vi "FT10_Wait Minimum Milliseconds.vi"(7 "Minimum ms wait":u32, 8 "error in (no error)":errorcluster, 11 "previous millisecond timer value in":u32) -> (0 "error out":errorcluster, 3 "millisecond timer value out":u32)   [LabVIEW 2015]
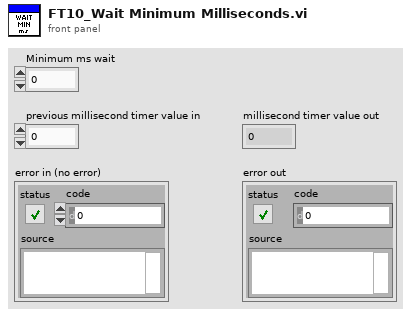
[diagram p1: front panel]
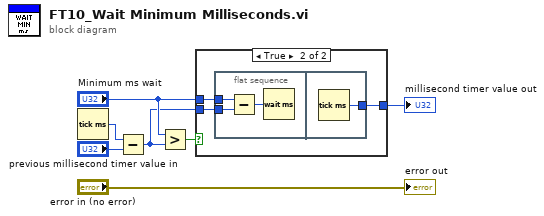
[diagram p0: block diagram]
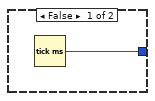
[diagram p2: hidden frame]
diagram:
  n1 = Tick Count (ms)() -> (millisecond timer value=w4:u32)
  n2 = Subtract(x=w4, y="previous millisecond timer value in") -> (x-y=w6:u32)
  n3 = Greater?(x="Minimum ms wait", y=w6) -> (0:w5:bool)
  n4 = case shown="True" w5 {
    tunnel: [w8 w11] -> w2
    tunnel: w6 -> [_ w9]
    tunnel: "Minimum ms wait" -> [_ w10]
    frame False {
      n5 = Tick Count (ms)() -> (millisecond timer value=w8:u32)
    }
    frame True {
      n6 = flat-sequence {
        tunnel: w10 -> [w14]
        tunnel: w9 -> [w13]
        tunnel: [w15] -> w11
        frame #0 {
          n7 = Subtract(x=w14, y=w13) -> (x-y=w12:u32)
          n8 = Wait (ms)(milliseconds to wait=w12) -> ()  [unwired: 1 out]
        }
        frame #1 {
          n9 = Tick Count (ms)() -> (millisecond timer value=w15:u32)
        }
      }
    }
  }
  "millisecond timer value out" <- w2
  "error out" <- "error in (no error)"
